vi "Get Most Recent Packages in Library.vi"(11 "LabVIEW Version (14.0)":string="14.0") -> (0 "error out":errorcluster, 2 "All VIPs in Library":T1[](array[typedef]), 3 "Varriant Attibute Table of newest Packages in Library":variant)   [LabVIEW 2017, in "CL_G3_VIPMUtilities.lvlib"]
doc: "Returns a variant lookup table of the newest vi packages added to the library. The key is the name and the value is the version number. The fullly qualified name is <name>-<number>."
uses:
  CL_G3_VIPMUtilities.lvlib
  <vilib>/JKI/VIPM API/command-line/support/Library Contents Cluster_vipm_api.ctl
  <vilib>/JKI/VIPM API/VIPM API_vipm_api.lvlib
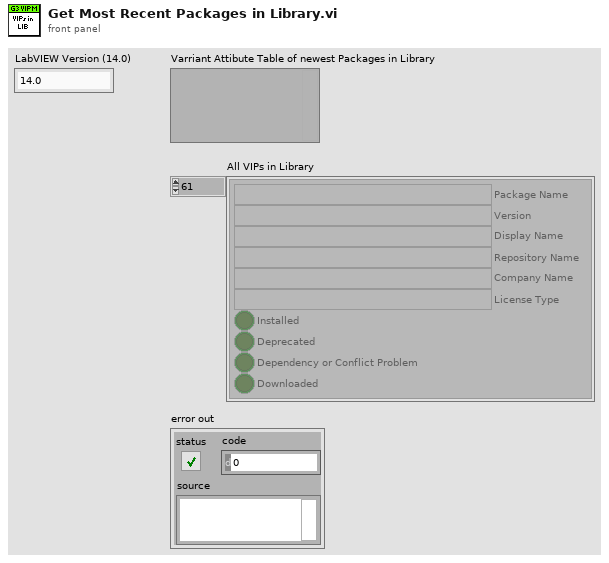
[diagram p1: front panel]
types:
  T1 = typedef "VIPM API_vipm_api.lvlib/Library Contents Cluster_vipm_api.ctl" = cluster{"Package Name":string, "Version":string, "Display Name":string, "Repository Name":string, "Company Name":string, "License Type":string, "Installed":bool, "Deprecated":bool, "Dependency or Conflict Problem":bool, "Downloaded":bool}
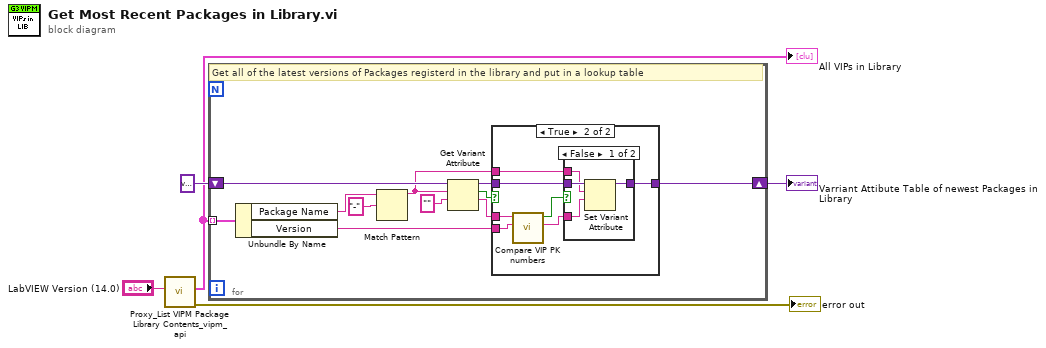
[diagram p0: block diagram]
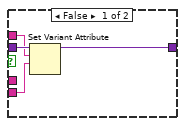
[diagram p2: hidden frame]
diagram:
  n1 = call "Proxy_List VIPM Package Library Contents_vipm_api.vi"("LabVIEW Version"="LabVIEW Version (14.0)") -> ("error out"=→"error out":errorcluster, "Library Contents []"=w2:T1[])  [unwired: 9 in]
  "All VIPs in Library" <- w2
  n2 = for {
    tunnel: w2 -> [w16] mode=indexing
    shift-right: [w15] -> w5
    shift-left: variant -> [w12]
    # "Get all of the latest versions of Packages registerd in the library and put in a lookup table"
    n3 = Unbundle By Name(w16) -> ("Package Name"=w14:string, "Version"=w6:string)
    n4 = Match Pattern(string=w14, regular expression="-") -> (before substring=w10:string)  [unwired: 1 in, 3 out]
    n5 = Get Variant Attribute(Variant=w12, name=w10, default value (empty Variant)="" ("regular expression")) -> (duplicate Variant=w11:variant, found=w7:bool, value=w8:string)  [unwired: 1 in, 1 out]
    n6 = case shown="True" w7 {
      tunnel: [w19 w27] -> w15
      tunnel: w11 -> [w20 w26]
      tunnel: w10 -> [w18 w25]
      tunnel: w8 -> [_ w24]
      tunnel: w6 -> [w17 w22]
      frame False {
        n7 = Set Variant Attribute(Variant=w20, name=w18, value=w17) -> (Variant out=w19:variant)  [unwired: 1 in, 2 out]
      }
      frame True {
        n8 = call "Compare VIP PK numbers.vi"("Y (#.#.#.#)"=w22, "X (#.#.#.#)"=w24) -> ("Largest"=w23:string, "X>Y"=w21:bool)  [unwired: 8 in]
        n9 = case shown="False" w21 {
          tunnel: [w31 w32] -> w27
          tunnel: w26 -> [w30 w32]
          tunnel: w25 -> [w29 _]
          tunnel: w23 -> [w28 _]
          frame False {
            n10 = Set Variant Attribute(Variant=w30, name=w29, value=w28) -> (Variant out=w31:variant)  [unwired: 1 in, 2 out]
          }
          frame True {
          }
        }
      }
    }
  }
  "Varriant Attibute Table of newest Packages in Library" <- w5
